vi "Write Config Data.vi"(0 "AI Channel":string, 1 "Sample Rate":dbl, 2 "Samples per Channel":i32, 3 "AO Channel":string, 5 "Error In":errorcluster) -> (14 "configuration file out":path, 19 "Error Out":errorcluster)   [LabVIEW 2019]
panel:
  # "Analog Input Channel Configuration"
  # "Analog Output Channel Configuration"
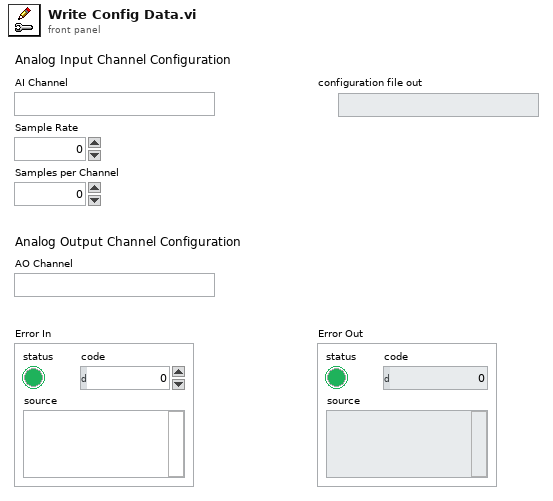
[diagram p1: front panel]
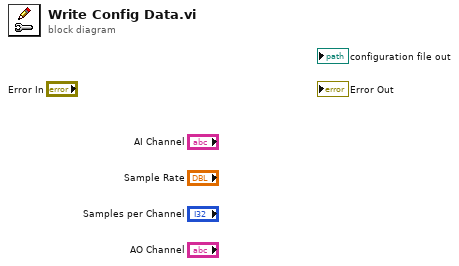
[diagram p0: block diagram]
diagram:
